vi "Carrier.vi"(9 "Phase":dbl, 10 "Carrier Frequency":dbl=10.1 caption="Frequency", 11 "Carrier Amplitude":dbl=1.0 caption="Amplitude") -> (2 "I(t) Carrier":waveform(dbl), 3 "R(t) Carrier":waveform(dbl))   [LabVIEW 2014]
uses:
  <vilib>/Analysis/NI_AALPro.lvlib
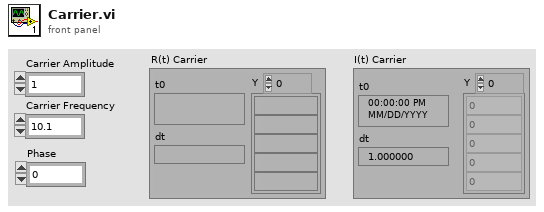
[diagram p1: front panel]
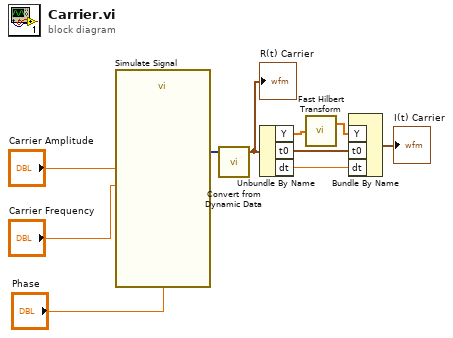
[diagram p0: block diagram]
diagram:
  n1 = call "Simulate Signal"("Frequency"="Carrier Frequency", "Amplitude"="Carrier Amplitude", "Phase"="Phase") -> ("Sine"=w8:dynamicdata)  [unwired: 11 in, 1 out]
  n2 = call "Convert from Dynamic Data"("Dynamic Data Type"=w8) -> ("Waveform"=w3:waveform(dbl))  [unwired: 3 in]
  "R(t) Carrier" <- w3
  n3 = Unbundle By Name(w3) -> ("Y"=w7:dbl[], "t0"=w6:timestamp, "dt"=w5:dbl)
  n4 = call <vilib>:"Fast Hilbert Transform.vi"("X"=w7) -> ("Hilbert{X}"=w4:dbl[])  [unwired: 1 out]
  n5 = Bundle By Name("Y"=w4, "t0"=w6, "dt"=w5) -> (→"I(t) Carrier":waveform(dbl))  [unwired: 1 in]
